vi "DPID.Create.vi"(8 "error in (no error)":errorcluster, 10 "DPID":T2, 11 "Section Ptr":T1 format="%.0x") -> (0 "error out":errorcluster, 3 "Parent Ref out":T1 format="%.0x")   [LabVIEW 2015, in "Diagnostics Addon System Explorer.lvlib"]
uses:
  Diagnostics Addon System Explorer.lvlib
  Types/DPID.Export.ctl
  Shared/Types/DPID.ctl
  Shared/Types/DPID.Rate.ctl
  <vilib>/NI Veristand/Custom Device API/Custom Device Item Ref.ctl
  Types/FG.Action.ctl
  ID.FG.vi
  <vilib>/NI Veristand/Custom Device API/NI VeriStand - Get Item Property.vi
  <vilib>/NI Veristand/Custom Device API/Get Item Property (U32 Array).vi
  <vilib>/NI Veristand/Custom Device API/Get Item Property (U32).vi
  <vilib>/NI/NI VeriStand Advanced SysDef API/SysDef API/SysDef.Property.Set.vi
  <vilib>/NI/NI VeriStand Advanced SysDef API/_SubVIs/SysDef.Property.Set.U32.vi
  Shared/SubVIs/Constants.vi
  <vilib>/NI/NI VeriStand Advanced SysDef API/_SubVIs/SysDef.Property.Set.U32.Array.vi
  Shared/Diagnostics Addon Shared.lvlib
  <vilib>/NI/NI VeriStand Advanced SysDef API/SysDef API/Advanced System Definition.lvlib
  <vilib>/NI VeriStand/Custom Device API/Custom Device API.lvlib
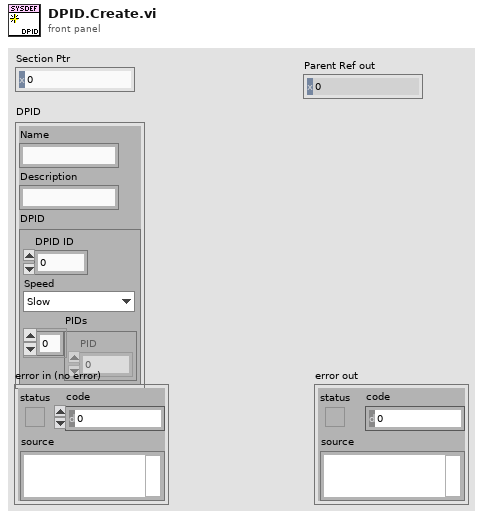
[diagram p1: front panel]
types:
  T1 = typedef "Custom Device API.lvlib/Custom Device Item Ref.ctl" = u64
  T2 = typedef "Diagnostics Addon System Explorer.lvlib/DPID.Export.ctl" = cluster{"Name":string, "Description":string, "DPID":T3}
  T3 = typedef "Diagnostics Addon Shared.lvlib/DPID.ctl" = cluster{"DPID ID":u8, "Speed":T4, "PIDs":u16[]}
  T4 = typedef "Diagnostics Addon Shared.lvlib/DPID.Rate.ctl" = enum16{"Slow", "Medium", "Fast"}
  T5 = typedef "Diagnostics Addon System Explorer.lvlib/FG.Action.ctl" = enum16{"Get", "Set"}
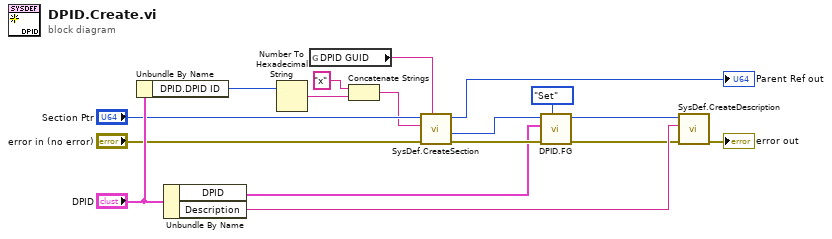
[diagram p0: block diagram]
diagram:
  n1 = Unbundle By Name("DPID") -> ("DPID.DPID ID"=w15:u8)
  n2 = Unbundle By Name("DPID") -> ("DPID"=w1:T3, "Description"=w8:string)
  n3 = Number To Hexadecimal String(2:w15) -> (0:w17:string)  [unwired: 1 in]
  n4 = global read "Constants.vi" "DPID GUID"() -> (w13:string)
  n5 = Concatenate Strings("x" ("string"), w17) -> (w10:string)
  n6 = call <vilib>:"SysDef.CreateSection.vi"("GUID"=w13, "error in (no error)"="error in (no error)", "Name"=w10, "nodeID"="Section Ptr") -> ("error out"=w6:errorcluster, "New NodeID"=w4:u64, "nodeID out"=→"Parent Ref out":u64)  [unwired: 4 in, 1 out]
  n7 = call "DPID.FG.vi"("Action"=FG.Action."Set", "error in (no error)"=w6, "DPID"=w1, "Device Item Ref in"=w4) -> ("error out"=w5:errorcluster, "Device Item Ref out"=w3:T1)  [unwired: 5 in, 1 out]
  n8 = call <vilib>:"SysDef.CreateDescription.vi"("error in (no error)"=w5, "Description"=w8, "ID in"=w3) -> ("error out"=→"error out":errorcluster)  [unwired: 7 in, 1 out]
